vi "FV_init_motor.vi"(8 "error in":errorcluster, 9 "velocity":dbl, 10 "steps_per_rev":i32=200, 11 "VISA in":refnum<visa-resource-name>) -> (0 "error out":errorcluster, 1 "motor_alarm":i32, 2 "motor_status":i32, 3 "VISA out":refnum<visa-resource-name>, 4 "status":bool, 5 "is_on":bool)   [LabVIEW 2019]
panel:
  # "If you change \"steps_per_rev\",\nsome other VIs have to be changed accordingly."
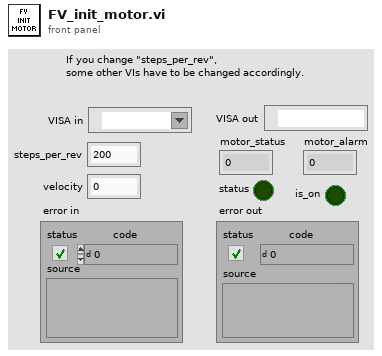
[diagram p1: front panel]
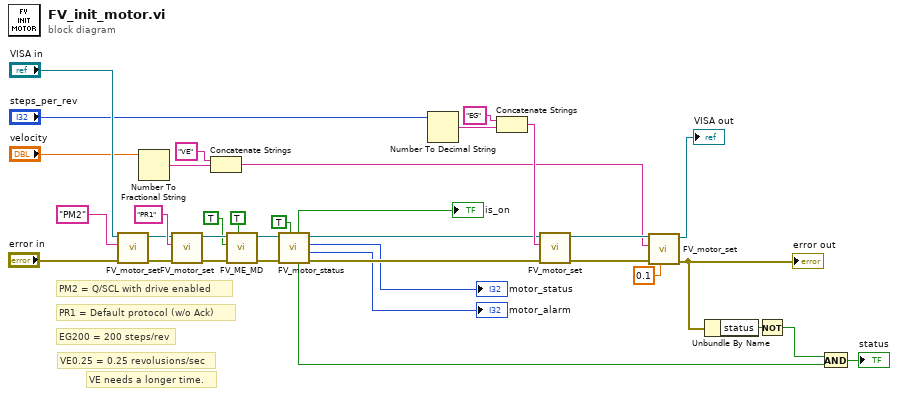
[diagram p0: block diagram]
diagram:
  # "VE needs a longer time."
  # "VE0.25 = 0.25 revolusions/sec"
  # "EG200 = 200 steps/rev"
  # "PR1 = Default protocol (w/o Ack)"
  # "PM2 = Q/SCL with drive enabled"
  n1 = call "FV_motor_set.vi"("error in"="error in", "command"="PM2", "VISA in"="VISA in") -> ("error out"=w17:errorcluster, "VISA out"=w24:refnum<visa-resource-name>)  [unwired: 7 in]
  n2 = Number To Fractional String(number="velocity") -> (F-format string=w25:string)  [unwired: 3 in]
  n3 = call "FV_motor_set.vi"("error in"=w17, "command"="PR1", "VISA in"=w24) -> ("error out"=w6:errorcluster, "VISA out"=w3:refnum<visa-resource-name>)  [unwired: 7 in]
  n4 = Concatenate Strings("VE", w25) -> (w21:string)
  n5 = call "FV_ME_MD.vi"("do_reset"=TRUE, "error in"=w6, "enable_or_disable"=TRUE, "VISA in"=w3) -> ("error out"=w5:errorcluster, "VISA out"=w4:refnum<visa-resource-name>)  [unwired: 5 in, 1 out]
  n6 = call "FV_motor_status.vi"("do_reset"=TRUE, "error in"=w5, "VISA"=w4) -> ("error out"=w13:errorcluster, "motor_alarm"=→"motor_alarm":i32, "motor_status"=→"motor_status":i32, "VISA out"=w14:refnum<visa-resource-name>, "status"=w9:bool, "is_on"=→"is_on":bool)  [unwired: 3 in]
  n7 = Number To Decimal String(number="steps_per_rev") -> (decimal integer string=w30:string)  [unwired: 1 in]
  n8 = Concatenate Strings("EG", w30) -> (w28:string)
  n9 = call "FV_motor_set.vi"("error in"=w13, "command"=w28, "VISA in"=w14) -> ("error out"=w16:errorcluster, "VISA out"=w23:refnum<visa-resource-name>)  [unwired: 7 in]
  n10 = call "FV_motor_set.vi"("delay  (sec)"=0.1, "error in"=w16, "command"=w21, "VISA in"=w23) -> ("error out"=w20:errorcluster, "VISA out"=→"VISA out":refnum<visa-resource-name>)  [unwired: 6 in]
  "error out" <- w20
  n11 = Unbundle By Name(w20) -> ("status"=w19:bool)
  n12 = Not(x=w19) -> (.not. x?=w18:bool)
  n13 = And(x=w18, y=w9) -> (x .and. y?=→"status":bool)
